vi "Global niWrite Lock.vi"() -> ()   [LabVIEW 2019]
panel:
  out "NI Write Lock":bool
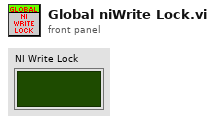
[diagram p1: front panel]
diagram:
